vi "ShrimpCam_Control.vi"() -> ()   [LabVIEW 2018]
panel:
  out "Gain 1'":i32
  out "Gain 2'":i32
  in  "Gain 2":i32
  in  "Gain 1":i32
  in  "base path 2":path=path "C:/Users/user/Shrimp_Data/Camera2"
  in  "base path 1":path=path "C:/Users/user/Shrimp_Data/Camera1"
  out "Framerate 2'":dbl
  out "Exposure time 2'":dbl
  in  "Exposure time 2":dbl=0.02
  in  "Framerate 2":dbl=15.0
  out "Image 2":picture
  out "Cam 2 Info":T1={"Bits/Pixel"=8, "Width"=8, "Height Height"=8, "Serial Number "=""}
  in  "Error In 2":errorcluster caption="Error In"
  in  "Camera 2 ID":i32
  out "Framerate 1'":dbl
  out "Exposure time 1'":dbl
  in  "Exposure time 1":dbl=0.02
  in  "Framerate 1":dbl=15.0
  out "Image 1":picture
  out "Cam 1  Info":T1={"Bits/Pixel"=8, "Width"=8, "Height Height"=8, "Serial Number "=""}
  in  "stop":bool
  in  "Error In 1":errorcluster caption="Error In"
  in  "Camera 1 ID":i32
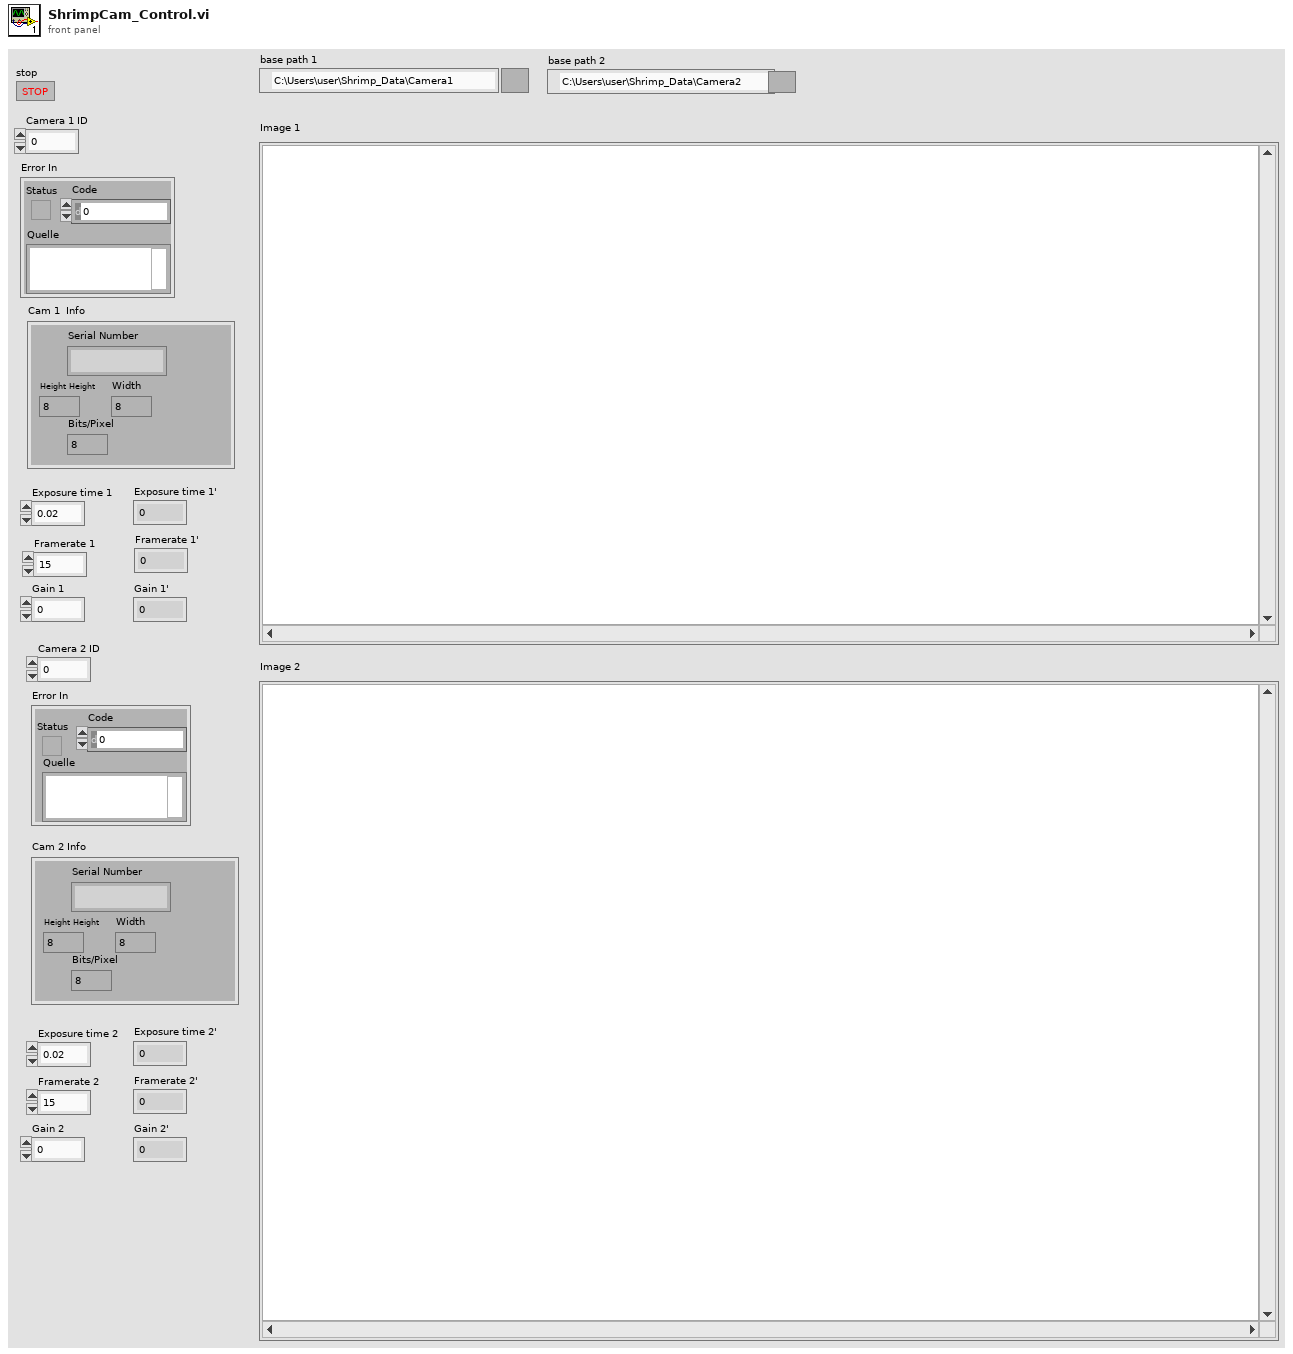
[diagram p1: front panel]
types:
  T1 = cluster{"Bits/Pixel":i32, "Width":i32, "Height Height":i32, "Serial Number ":string}
  T2 = typedef "imagedata.ctl" = cluster{"image type":i32, "image depth":i32, "image":u8[], "mask":u8[], "colors":u32[], "Rectangle":cluster{"left":i16, "top":i16, "right":i16, "bottom":i16}}
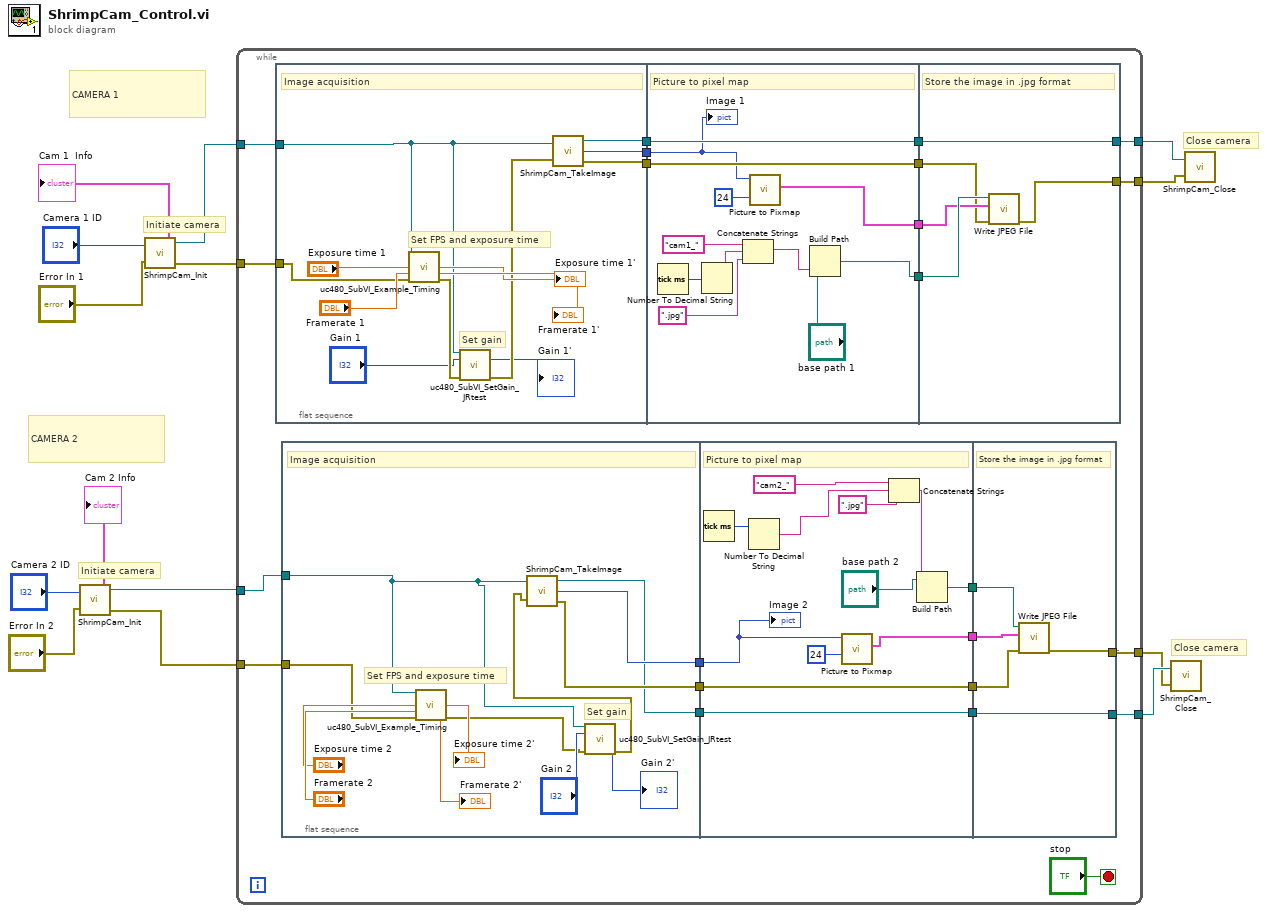
[diagram p0: block diagram]
diagram:
  # "Initiate camera"
  # "Close camera"
  # "CAMERA 1"
  # "CAMERA 2"
  # "Close camera"
  # "Initiate camera"
  n1 = call "ShrimpCam_Init.vi"("Camera ID"="Camera 2 ID", "Error In"="Error In 2") -> ("Ref (cam out)"=w6:refnum<k24>, "Cam Info"=→"Cam 2 Info":T1, "Error Out"=w7:errorcluster)
  n2 = call "ShrimpCam_Init.vi"("Camera ID"="Camera 1 ID", "Error In"="Error In 1") -> ("Ref (cam out)"=w12:refnum<k24>, "Cam Info"=→"Cam 1  Info":T1, "Error Out"=w5:errorcluster)
  n3 = while {
    tunnel: w12 -> [w36]
    tunnel: w7 -> [w35]
    tunnel: w6 -> [w15]
    tunnel: [w34] -> w4
    tunnel: w5 -> [w33]
    tunnel: [w32] -> w2
    tunnel: [w31] -> w1
    tunnel: [w23] -> w3
    stop <- "stop" stop-if-true
    n4 = flat-sequence {
      tunnel: w36 -> [w70]
      tunnel: [w78] -> w22
      tunnel: w33 -> [w75]
      tunnel: [w73] -> w20
      tunnel: [w72] -> w18
      tunnel: w22 -> [w92]
      tunnel: [w92] -> w21
      tunnel: w20 -> [w91]
      tunnel: [w91] -> w19
      tunnel: w18 -> [w81]
      tunnel: [w85] -> w17
      tunnel: [w84] -> w16
      tunnel: w21 -> [w93]
      tunnel: w19 -> [w94]
      tunnel: [w93] -> w32
      tunnel: [w97] -> w31
      tunnel: w17 -> [w96]
      tunnel: w16 -> [w95]
      frame #0 {
        # "Set gain"
        # "Set FPS and exposure time"
        # "Image acquisition"
        n5 = call "uc480_SubVI_Example_Timing.vi"(".NET (Reference)"=w70, "Exposure time"="Exposure time 1", "Framerate"="Framerate 1", "Error In"=w75) -> ("Exposure time"=→"Exposure time 1'":dbl, "Framerate"=→"Framerate 1'":dbl, "Error Out"=w74:errorcluster)  [unwired: 8 in, 1 out]
        n6 = call "uc480_SubVI_SetGain_JRtest.vi"(".NET (Reference)"=w70, "Gain"="Gain 1", "Error In"=w74) -> ("Gain (out)"=→"Gain 1'":i32, "Error Out"=w71:errorcluster)  [unwired: 11 in]
        n7 = call "ShrimpCam_TakeImage.vi"("Ref (cam in)"=w70, "Error In"=w71) -> ("Ref (cam out)"=w78:refnum<k24>, "Image"=w72:picture, "Error Out"=w73:errorcluster)
      }
      frame #1 {
        # "Picture to pixel map"
        n8 = Tick Count (ms)() -> (millisecond timer value=w89:u32)
        n9 = Number To Decimal String(number=w89) -> (decimal integer string=w83:string)  [unwired: 1 in]
        n10 = Concatenate Strings("cam1_", w83, ".jpg" ("string")) -> (w88:string)
        n11 = call <vilib>:"Picture to Pixmap.vi"("depth"=24, "picture"=w81) -> ("image data"=w84:T2)  [unwired: 8 in, 1 out]
        n12 = Build Path(base path="base path 1", name or relative path=w88) -> (appended path=w85:path)
        "Image 1" <- w81
      }
      frame #2 {
        # "Store the image in .jpg format"
        n13 = call <vilib>:"Write JPEG File.vi"("error in (no error)"=w94, "image data"=w95, "path to JPEG file"=w96) -> ("error out"=w97:errorcluster)  [unwired: 7 in, 1 out]
      }
    }
    n14 = flat-sequence {
      tunnel: [w50] -> w30
      tunnel: w35 -> [w45]
      tunnel: [w44] -> w29
      tunnel: [w43] -> w27
      tunnel: w15 -> [w39]
      tunnel: w30 -> [w62]
      tunnel: w29 -> [w61]
      tunnel: [w61] -> w28
      tunnel: w27 -> [w60]
      tunnel: [w60] -> w26
      tunnel: [w56] -> w25
      tunnel: [w58] -> w24
      tunnel: w28 -> [w65]
      tunnel: [w67] -> w34
      tunnel: w26 -> [w67]
      tunnel: w25 -> [w66]
      tunnel: w24 -> [w63]
      tunnel: [w64] -> w23
      frame #0 {
        # "Set gain"
        # "Set FPS and exposure time"
        # "Image acquisition"
        n15 = call "uc480_SubVI_Example_Timing.vi"(".NET (Reference)"=w39, "Exposure time"="Exposure time 2", "Framerate"="Framerate 2", "Error In"=w45) -> ("Exposure time"=→"Exposure time 2'":dbl, "Framerate"=→"Framerate 2'":dbl, "Error Out"=w41:errorcluster)  [unwired: 8 in, 1 out]
        n16 = call "uc480_SubVI_SetGain_JRtest.vi"(".NET (Reference)"=w39, "Gain"="Gain 2", "Error In"=w41) -> ("Gain (out)"=→"Gain 2'":i32, "Error Out"=w40:errorcluster)  [unwired: 11 in]
        n17 = call "ShrimpCam_TakeImage.vi"("Ref (cam in)"=w39, "Error In"=w40) -> ("Ref (cam out)"=w43:refnum<k24>, "Image"=w50:picture, "Error Out"=w44:errorcluster)
      }
      frame #1 {
        # "Picture to pixel map"
        n18 = Tick Count (ms)() -> (millisecond timer value=w55:u32)
        n19 = Number To Decimal String(number=w55) -> (decimal integer string=w54:string)  [unwired: 1 in]
        n20 = call <vilib>:"Picture to Pixmap.vi"("depth"=24, "picture"=w62) -> ("image data"=w58:T2)  [unwired: 8 in, 1 out]
        n21 = Concatenate Strings("cam2_" ("string"), w54, ".jpg" ("string")) -> (w57:string)
        n22 = Build Path(base path="base path 2", name or relative path=w57) -> (appended path=w56:path)
        "Image 2" <- w62
      }
      frame #2 {
        # "Store the image in .jpg format"
        n23 = call <vilib>:"Write JPEG File.vi"("error in (no error)"=w65, "image data"=w63, "path to JPEG file"=w66) -> ("error out"=w64:errorcluster)  [unwired: 7 in, 1 out]
      }
    }
  }
  n24 = call "ShrimpCam_Close.vi"("Error In"=w3, "Ref (cam in)"=w4) -> ()  [unwired: 1 in, 1 out]
  n25 = call "ShrimpCam_Close.vi"("Error In"=w1, "Ref (cam in)"=w2) -> ()  [unwired: 1 in, 1 out]
